vi "Get Next Step.vi"(8 "error in (no error)":errorcluster, 11 "Sequencer in":refnum<class "Sequencer.lvclass">) -> (0 "error out":errorcluster, 1 "Parameter":variant, 2 "Step":string, 3 "Sequencer out":refnum<class "Sequencer.lvclass">, 4 "Reply Channel":refnum<notifier>)   [LabVIEW 2015, in "Sequencer.lvclass"]
uses:
  Sequencer.lvclass
  Messaging/Message/Message.lvclass
  Sequencer.lvclass/Sequencer.ctl
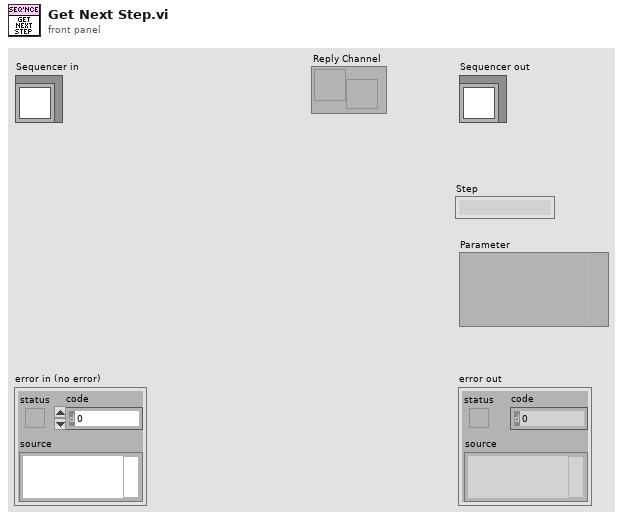
[diagram p1: front panel]
types:
  T1 = typedef "Sequencer.lvclass/Single Step Data.ctl" = cluster{"Step":string, "Parameter":variant, "Reply Channel":refnum<notifier>}
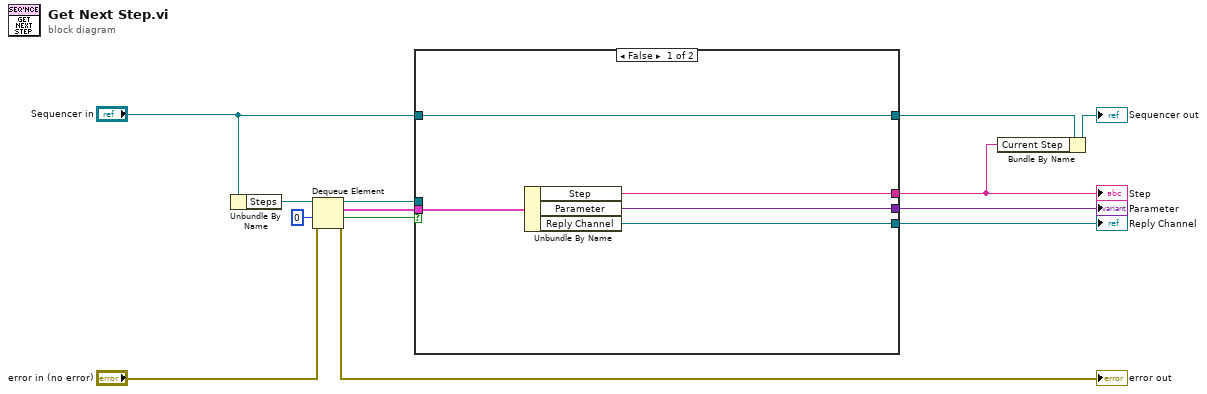
[diagram p0: block diagram]
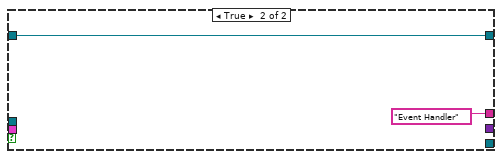
[diagram p2: hidden frame]
diagram:
  n1 = Unbundle By Name("Sequencer in") -> ("Steps"=w1:refnum<queue>)
  n2 = Dequeue Element(queue=w1, timeout in ms (-1)=0, error in (no error)="error in (no error)") -> (queue out=w5:refnum<queue>, element=w2:T1, timed out?=w3:bool, error out=→"error out":errorcluster)
  n3 = case shown="False" w3 {
    tunnel: "Sequencer in" -> [w17 w20]
    tunnel: [w17 w20] -> w8
    tunnel: [w16 "Event Handler" ("String")] -> w7
    tunnel: [w15 _] -> w10
    tunnel: [w14 _] -> w6
    tunnel: w5 -> [_ _]
    tunnel: w2 -> [w18 _]
    frame False {
      n4 = Unbundle By Name(w18) -> ("Step"=w16:string, "Parameter"=w15:variant, "Reply Channel"=w14:refnum<notifier>)
    }
    frame True {
    }
  }
  "Step" <- w7
  "Parameter" <- w10
  "Reply Channel" <- w6
  n5 = Bundle By Name(cluster=w8, "Current Step"=w7) -> (→"Sequencer out":refnum<class "Sequencer.lvclass">)
